vi "Open Dir.vi"(8 "error in":errorcluster, 10 "dir":string, 11 "path":path) -> (0 "error out":errorcluster)   [LabVIEW 2015]
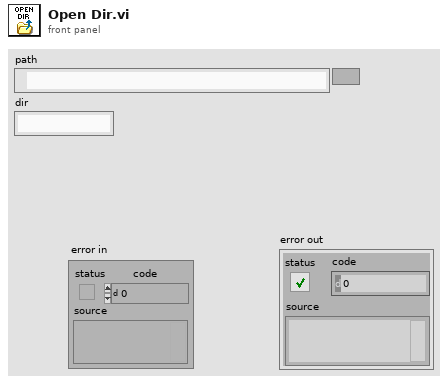
[diagram p1: front panel]
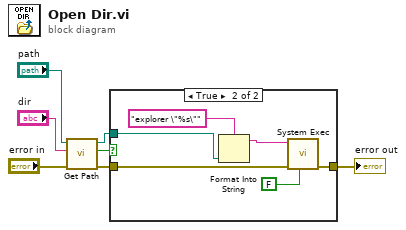
[diagram p0: block diagram]
diagram:
  n1 = call "Get Path.vi"("error in"="error in", "dir"="dir", "path"="path") -> ("error out"=w3:errorcluster, "file or folder exists?"=w5:bool, "dup path"=w6:path)  [unwired: 6 in]
  n2 = case shown="True" w5 {
    tunnel: w3 -> [w8 w12]
    tunnel: [w8 w11] -> w7
    tunnel: w6 -> [_ w9]
    frame False {
    }
    frame True {
      n3 = Format Into String(format string="explorer \"%s\"", w9) -> (resulting string=w10:string)  [unwired: 2 in, 1 out]
      n4 = call <vilib>:"System Exec.vi"("run minimized? (F)"=FALSE, "error in (no error)"=w12, "command line"=w10) -> ("error out"=w11:errorcluster)  [unwired: 5 in, 3 out]
    }
  }
  "error out" <- w7
